vi "ProfiledPIDController_Execute.vi"(4 "PID Error Tolerance":T3={"PositionTolerance"=0.001, "VelocityTolerance"=9.9e+30}, 5 "Constraints":T1 {"MaxAcceleration" format="%16_6e"; "MaxVelocity" format="%16_6e"}, 6 "Period":dbl=0.02, 7 "PID Input Limits":T2, 8 "Reset":bool, 9 "SP-SetPoint Goal":dbl, 10 "PV-Measurement":dbl, 11 "PID Tuning":T4={"Kp"=0.0, "Ki"=0.0, "Kd"=0.0, "MaximumIntegral"=9.9e+30, "MinimumIntegral"=-9.9e+30}) -> (0 "out PID_CONTROLLER":T5={"Controller"={"Kp"=0.0, "Ki"=0.0, "Kd"=0.0, "Period"=0.0, "Max_Integral"=1.0, "Min_Integral"=-1.0, "Max_Input"=0.0, "Min_Input"=0.0, "Continuous"=FALSE, "PositionError"=0.0, "VelocityError"=0.0, "PrevError"=0.0, "TotalError"=0.0, "PositionTolerance"=0.05, "VelocityTolerance"=9.99e+35, "SetPoint"=0.0, "Kf"=0.0, "Prev_Deriv"=0.0, "Prev_Deriv 2"=0.0, "DerivativeFilter"=FALSE, "Min_Output"=-9.99e+35, "Max_Output"=9.9e+35, "Prev_F_P"=0.0, "Prev_F_P_2"=0.0, "AntiWindupActive"=FALSE, "Measurement"=0.0}, "Goal"={"Position"=0.0, "Velocity"=0.0}, "Setpoint"={"Position"=0.0, "Velocity"=0.0}, "Constraint"={"MaxVelocity"=0.0, "MaxAcceleration"=0.0}} {"Constraint"."MaxAcceleration" format="%16_6e"; "Constraint"."MaxVelocity" format="%16_6e"; "Setpoint"."Velocity" format="%16_6e"; "Setpoint"."Position" format="%16_6e"; "Goal"."Velocity" format="%16_6e"; "Goal"."Position" format="%16_6e"; "Controller"."Measurement" format="%16_6e"; "Controller"."Prev_F_P_2" format="%16_6e"; "Controller"."Prev_F_P" format="%16_6e"; "Controller"."Max_Output" format="%16_6e"; "Controller"."Min_Output" format="%16_6e"; "Controller"."Prev_Deriv 2" format="%16_6e"; "Controller"."Prev_Deriv" format="%16_6e"; "Controller"."Kf" format="%16_6e"; "Controller"."SetPoint" format="%16_6e"; "Controller"."VelocityTolerance" format="%16_6e"; "Controller"."PositionTolerance" format="%16_6e"; "Controller"."TotalError" format="%16_6e"; "Controller"."PrevError" format="%16_6e"; "Controller"."VelocityError" format="%16_6e"; "Controller"."PositionError" format="%16_6e"; "Controller"."Min_Input" format="%16_6e"; "Controller"."Max_Input" format="%16_6e"; "Controller"."Min_Integral" format="%16_6e"; "Controller"."Max_Integral" format="%16_6e"; "Controller"."Period" format="%16_6e"; "Controller"."Kd" format="%16_6e"; "Controller"."Ki" format="%16_6e"; "Controller"."Kp" format="%16_6e"}, 1 "AtSetpoint":bool, 2 "AtGoal":bool, 3 "CO-ControlOutput":dbl)   [LabVIEW 2019, in "Trajectory_Library.lvlib"]
doc: "Convience, single call, LabVIEW function. Creates and calculates the Profiled PID controller. Call this routine periodically to calculate the newest output for the provided inputs. \n \nInputs:\n - Constraints -- Trapezoid Constraint cluster contains\n - Maximum Velocity\n - Maximum Accleration\n - PID Input Limits -- (Optional) Cluster containing:\n - MaxInput -- (Default: 0)\n - MinInput -- (Default: 0)\n - Continous -- When True indicates that the input is continuous. (Default: False)\n - PID Tuning -- PID Tuning parameters containing:\n - Kp -- The proportional coefficient.\n - Ki -- The integral coefficient.\n - Kd -- The derivative coefficient.\n - Maximum Integral -- The maximum value of the integrator.\n - Minimum Integral -- The minimum value of the integrator.\n - PV-measurement -- The current measurement of the process variable. (PV)\n - SP-setpoint goal -- The new end goal setpoint of the controller. (SP)\n - Reset -- When True, causes the PID to be reset. (Default: False)\n - Period -- Period of repeated calls in seconds. (Default: 0.020)\n - PID Error Tolerance -- Tolerances for determining \"At Setpoint\", contains:\n - Position Tolerance -- (Default: 0.001)\n - Velocity Tolerance -- (Default: 9.9E+30)\nOutputs:\n - CO-ControlOutput -- Controller output (CO) \n - AtGoal -- True when PV is within the specified tolerances of the final goal SP.\n - AtSetpoint -- True when PV is within the specified tolerances of the internediate position SP.\n - Profield PID_Controller -- Updated PID_Controller data cluster"
uses:
  Trajectory_Library.lvlib
  TypeDef/PID_CONTROLLER.ctl
  TypeDef/PID_TUNING.ctl
  TypeDef/PID_INPUT_LIMITS.ctl
  TypeDef/PID_ERROR_TOLERANCE.ctl
  TypeDef/TRAPEZOID_PROFILE_STATE.ctl
  TypeDef/TRAPEZOID_PROFILE_CONSTRAINT.ctl
  TypeDef/PROFILED_PID_CONTROLLER.ctl
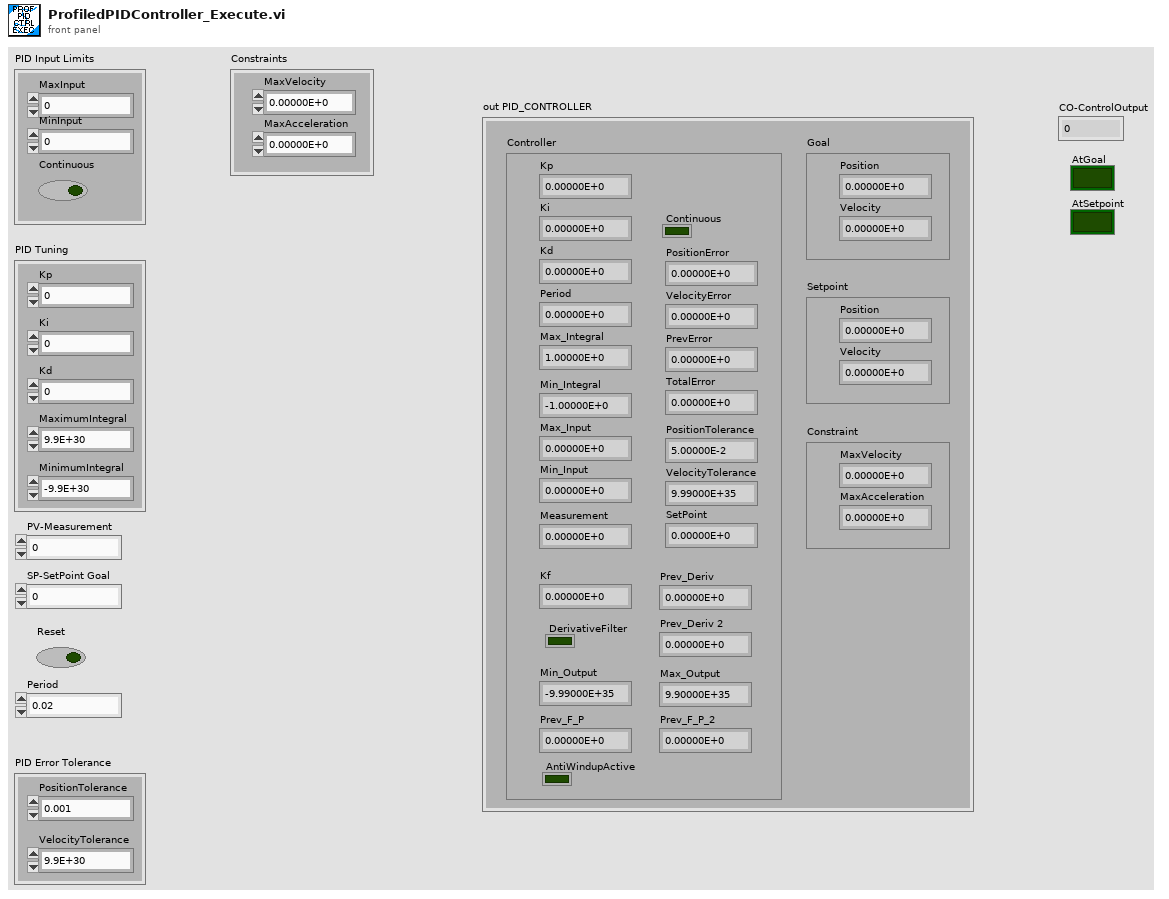
[diagram p1: front panel]
types:
  T1 = typedef "Trajectory_Library.lvlib/TRAPEZOID_PROFILE_CONSTRAINT.ctl" = cluster{"MaxVelocity":dbl, "MaxAcceleration":dbl}
  T2 = typedef "Trajectory_Library.lvlib/PID_INPUT_LIMITS.ctl" = cluster{"MaxInput":dbl, "MinInput":dbl, "Continuous":bool}
  T3 = typedef "Trajectory_Library.lvlib/PID_ERROR_TOLERANCE.ctl" = cluster{"PositionTolerance":dbl, "VelocityTolerance":dbl}
  T4 = typedef "Trajectory_Library.lvlib/PID_TUNING.ctl" = cluster{"Kp":dbl, "Ki":dbl, "Kd":dbl, "MaximumIntegral":dbl, "MinimumIntegral":dbl}
  T5 = typedef "Trajectory_Library.lvlib/PROFILED_PID_CONTROLLER.ctl" = cluster{"Controller":T6, "Goal":T7, "Setpoint":T7, "Constraint":T1}
  T6 = typedef "Trajectory_Library.lvlib/PID_CONTROLLER.ctl" = cluster{"Kp":dbl, "Ki":dbl, "Kd":dbl, "Period":dbl, "Max_Integral":dbl, "Min_Integral":dbl, "Max_Input":dbl, "Min_Input":dbl, "Continuous":bool, "PositionError":dbl, "VelocityError":dbl, "PrevError":dbl, "TotalError":dbl, "PositionTolerance":dbl, "VelocityTolerance":dbl, "SetPoint":dbl, "Kf":dbl, "Prev_Deriv":dbl, "Prev_Deriv 2":dbl, "DerivativeFilter":bool, "Min_Output":dbl, "Max_Output":dbl, "Prev_F_P":dbl, "Prev_F_P_2":dbl, "AntiWindupActive":bool, "Measurement":dbl}
  T7 = typedef "Trajectory_Library.lvlib/TRAPEZOID_PROFILE_STATE.ctl" = cluster{"Position":dbl, "Velocity":dbl}
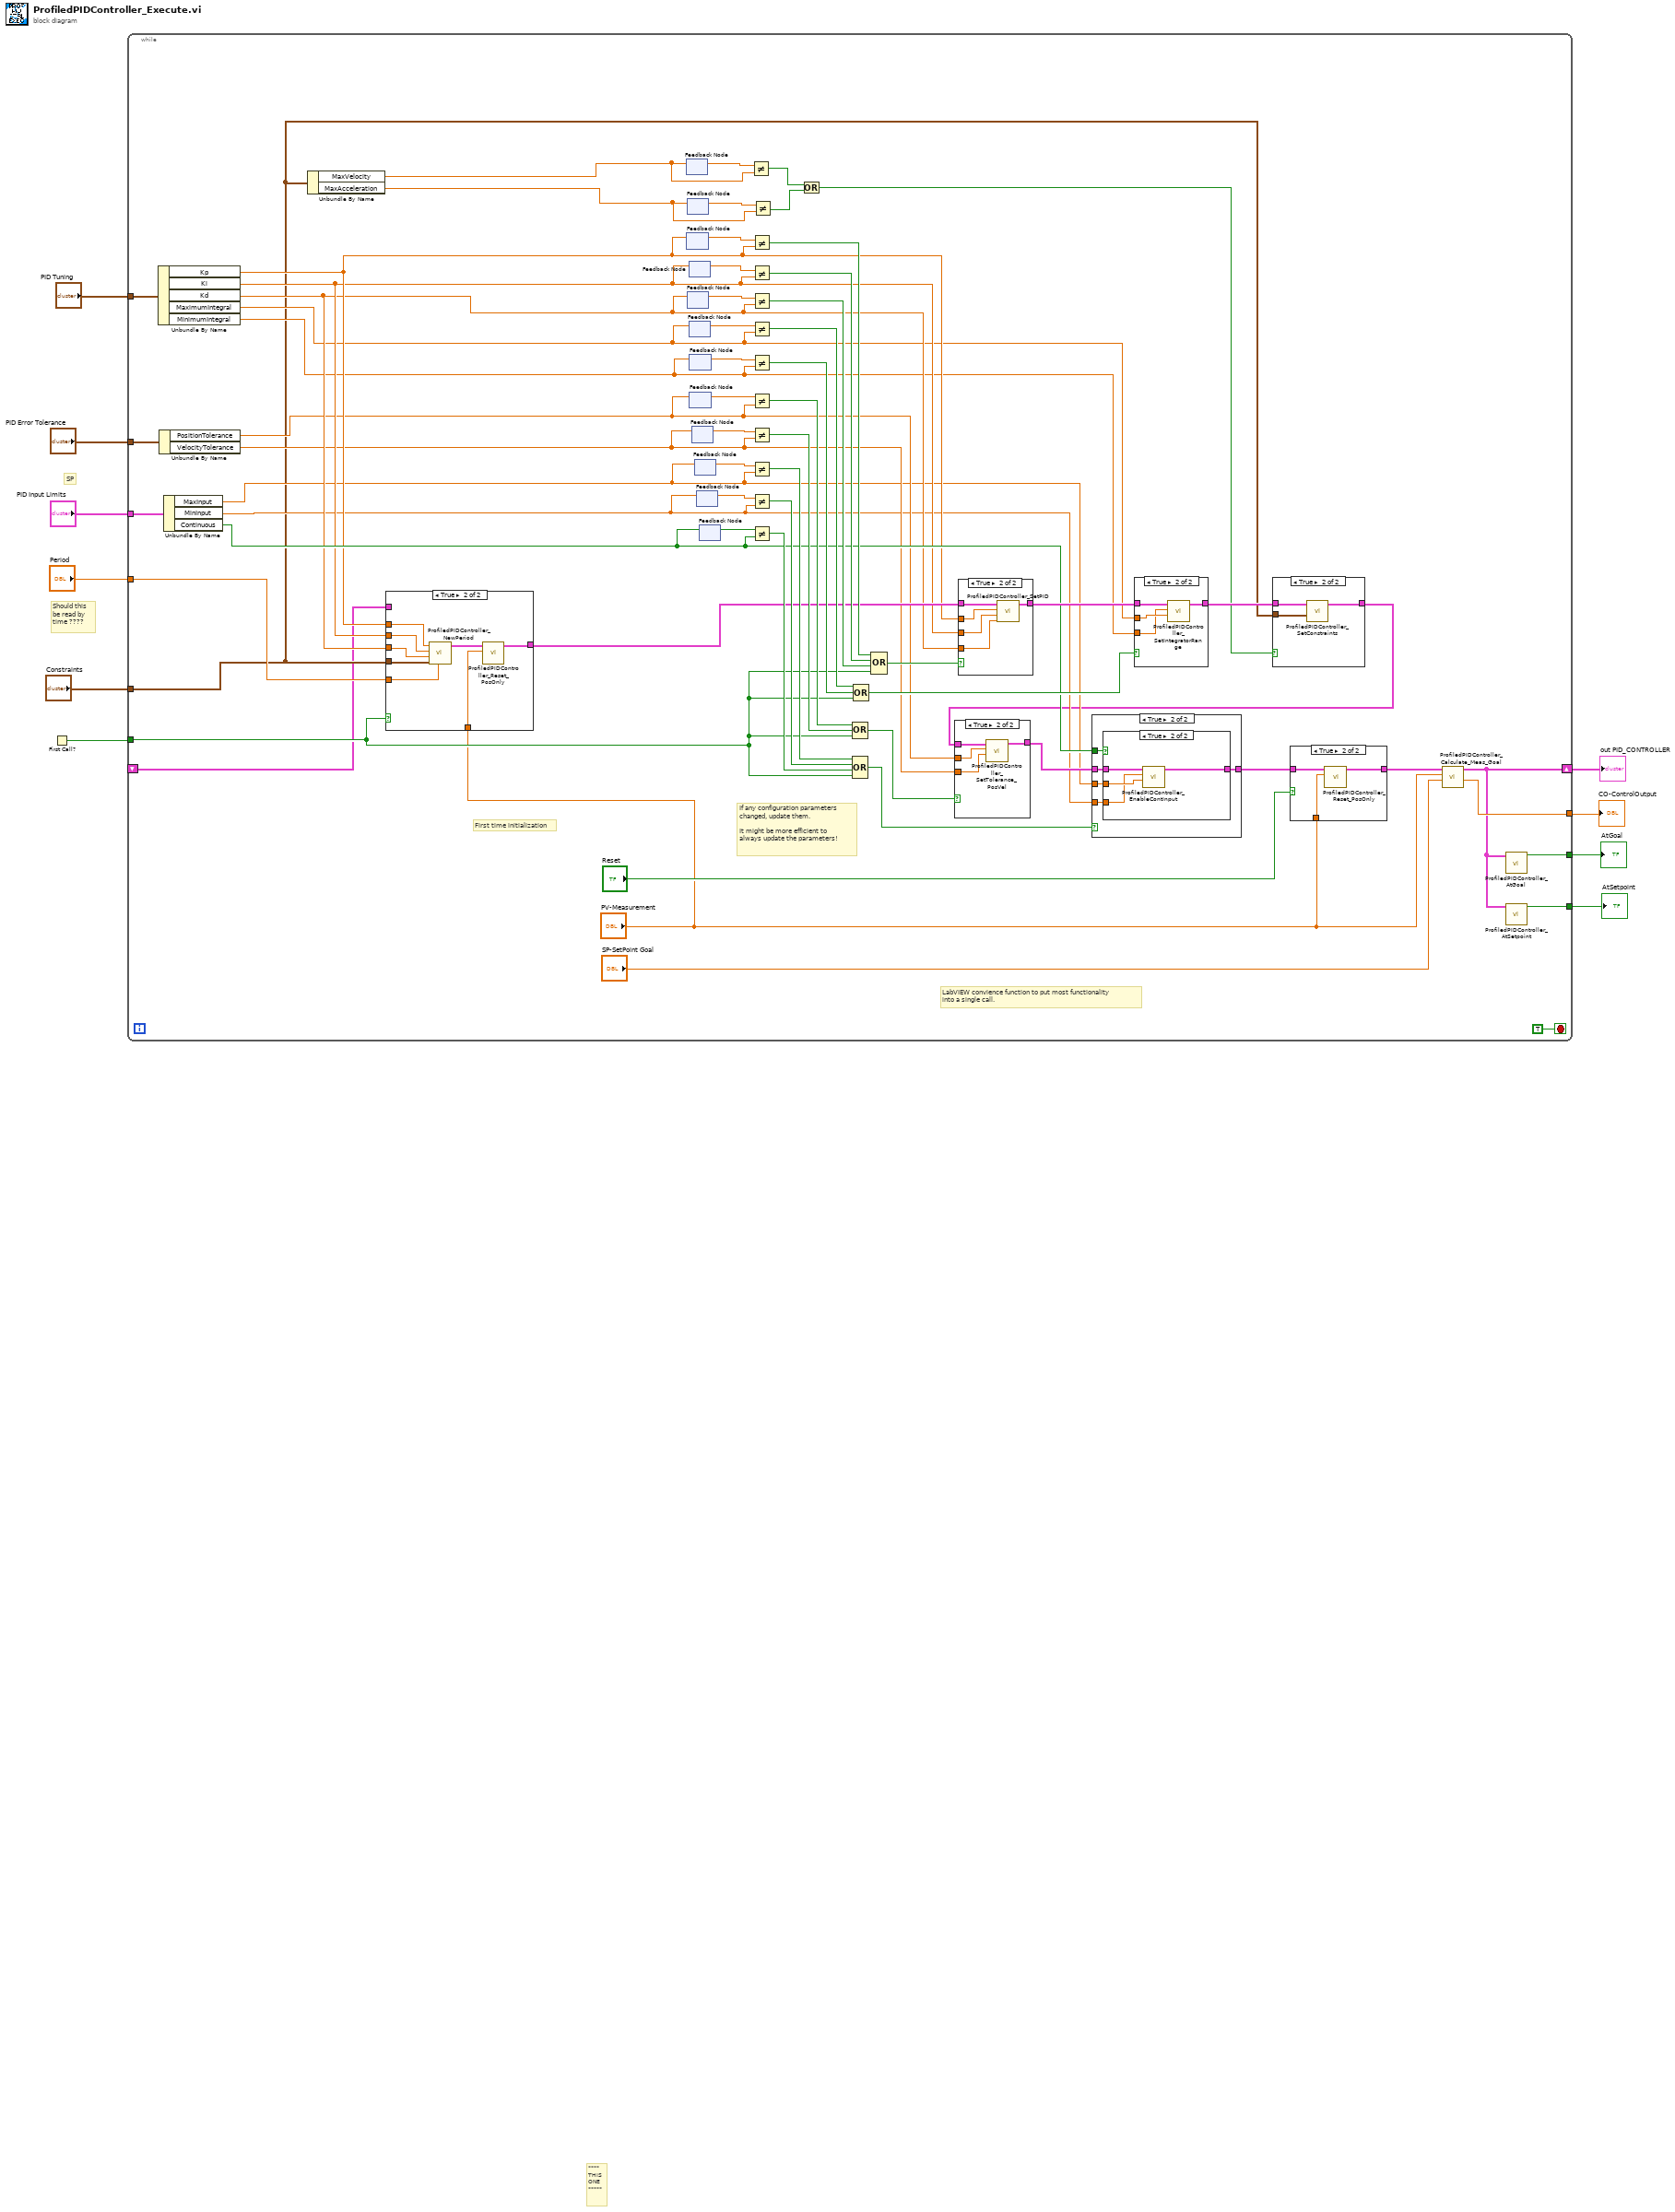
[diagram p0: block diagram]
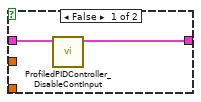
[diagram p6: hidden frame]
diagram:
  # "Should this\nbe read by\ntime ????"
  # "SP"
  # "****\nTHIS\nONE\n*****"
  n1 = First Call?() -> (First Call?: T/F=w4:bool)
  n2 = while {
    tunnel: [w73] -> w10
    tunnel: "PID Tuning" -> [w71]
    tunnel: [w70] -> w8
    tunnel: "PID Error Tolerance" -> [w69]
    tunnel: "PID Input Limits" -> [w68]
    tunnel: "Period" -> [w66]
    tunnel: w4 -> [w26]
    tunnel: [w24] -> w3
    tunnel: "Constraints" -> [w13]
    shift-right: [w23] -> w2
    shift-left: _ -> [w12]
    stop <- TRUE stop-if-true
    # "First time initialization"
    # "If any configuration parameters \nchanged, update them.\n\nIt might be more efficient to\nalways update the parameters!"
    # "LabVIEW convience function to put most functionality\ninto a single call."
    n3 = Unbundle By Name(w71) -> ("Kp"=w44:dbl, "Ki"=w43:dbl, "Kd"=w42:dbl, "MaximumIntegral"=w41:dbl, "MinimumIntegral"=w40:dbl)
    n4 = Unbundle By Name(w69) -> ("PositionTolerance"=w39:dbl, "VelocityTolerance"=w38:dbl)
    n5 = Unbundle By Name(w68) -> ("MaxInput"=w37:dbl, "MinInput"=w36:dbl, "Continuous"=w46:bool)
    n6 = Unbundle By Name(w13) -> ("MaxVelocity"=w17:dbl, "MaxAcceleration"=w18:dbl)
    n7 = case shown="True" w26 {
      tunnel: w44 -> [_ w86]
      tunnel: w43 -> [_ w85]
      tunnel: w42 -> [_ w84]
      tunnel: w66 -> [_ w83]
      tunnel: [w78 w80] -> w47
      tunnel: w12 -> [w78 _]
      tunnel: w13 -> [_ w81]
      tunnel: "PV-Measurement" -> [_ w79]
      frame False {
      }
      frame True {
        n8 = call "ProfiledPIDController_NewPeriod.vi"("Period"=w83, "Constraints"=w81, "Kd"=w84, "Ki"=w85, "Kp"=w86) -> ("PROFILED_PID_CONTROLLER"=w82:T5)  [unwired: 6 in]
        n9 = call "ProfiledPIDController_Reset_PosOnly.vi"("Position"=w79, "in PROFILED_PID_CONTROLLER"=w82) -> ("out PROFILED_PID_CONTROLLER"=w80:T5)  [unwired: 9 in]
      }
    }
    n10 = feedback #1() -> (w19:dbl)  [unwired: 1 in]
    n11 = feedback-in #1(w17) -> ()
    n12 = feedback #2() -> (w35:dbl)  [unwired: 1 in]
    n13 = feedback-in #2(w44) -> ()
    n14 = feedback #3() -> (w22:dbl)  [unwired: 1 in]
    n15 = feedback-in #3(w18) -> ()
    n16 = feedback #4() -> (w33:dbl)  [unwired: 1 in]
    n17 = feedback-in #4(w42) -> ()
    n18 = feedback #5() -> (w34:dbl)  [unwired: 1 in]
    n19 = feedback-in #5(w43) -> ()
    n20 = feedback #6() -> (w32:dbl)  [unwired: 1 in]
    n21 = feedback-in #6(w41) -> ()
    n22 = feedback #7() -> (w31:dbl)  [unwired: 1 in]
    n23 = feedback-in #7(w40) -> ()
    n24 = feedback #8() -> (w30:dbl)  [unwired: 1 in]
    n25 = feedback-in #8(w39) -> ()
    n26 = feedback #9() -> (w29:dbl)  [unwired: 1 in]
    n27 = feedback-in #9(w38) -> ()
    n28 = feedback #10() -> (w28:dbl)  [unwired: 1 in]
    n29 = feedback-in #10(w37) -> ()
    n30 = feedback #11() -> (w27:dbl)  [unwired: 1 in]
    n31 = feedback-in #11(w36) -> ()
    n32 = feedback #12() -> (w45:bool)  [unwired: 1 in]
    n33 = feedback-in #12(w46) -> ()
    n34 = Not Equal?(x=w19, y=w17) -> (x != y?=w16:bool)
    n35 = Not Equal?(x=w35, y=w44) -> (x != y?=w56:bool)
    n36 = Not Equal?(x=w34, y=w43) -> (x != y?=w57:bool)
    n37 = Not Equal?(x=w33, y=w42) -> (x != y?=w58:bool)
    n38 = Not Equal?(x=w32, y=w41) -> (x != y?=w59:bool)
    n39 = Not Equal?(x=w31, y=w40) -> (x != y?=w60:bool)
    n40 = Not Equal?(x=w30, y=w39) -> (x != y?=w61:bool)
    n41 = Not Equal?(x=w29, y=w38) -> (x != y?=w62:bool)
    n42 = Not Equal?(x=w28, y=w37) -> (x != y?=w63:bool)
    n43 = Not Equal?(x=w27, y=w36) -> (x != y?=w64:bool)
    n44 = Not Equal?(x=w45, y=w46) -> (x != y?=w65:bool)
    n45 = Not Equal?(x=w22, y=w18) -> (x != y?=w15:bool)
    n46 = Or(x=w16, y=w15) -> (x .or. y?=w14:bool)
    n47 = Compound Arithmetic op=OR(w61, w62, w26) -> (w52:bool)
    n48 = Compound Arithmetic op=OR(w63, w64, w65, w26) -> (w51:bool)
    n49 = Compound Arithmetic op=OR(w59, w60, w26) -> (w53:bool)
    n50 = Compound Arithmetic op=OR(w56, w57, w58, w26) -> (w55:bool)
    n51 = case shown="True" w55 {
      tunnel: w47 -> [w113 w118]
      tunnel: w44 -> [_ w117]
      tunnel: w43 -> [_ w116]
      tunnel: w42 -> [_ w115]
      tunnel: [w113 w114] -> w54
      frame False {
      }
      frame True {
        n52 = call "ProfiledPIDController_SetPID.vi"("Kd"=w115, "Ki"=w116, "Kp"=w117, "in PROFILED_PID_CONTROLLER"=w118) -> ("out PROFILED_PID_CONTROLLER"=w114:T5)  [unwired: 7 in]
      }
    }
    n53 = case shown="True" w53 {
      tunnel: w54 -> [w108 w112]
      tunnel: w41 -> [_ w111]
      tunnel: w40 -> [_ w110]
      tunnel: [w108 w109] -> w21
      frame False {
      }
      frame True {
        n54 = call "ProfiledPIDController_SetIntegratorRange.vi"("Maximum"=w111, "Minimum"=w110, "in PROFILED_PID_CONTROLLER"=w112) -> ("out PROFILED_PID_CONTROLLER"=w109:T5)  [unwired: 8 in]
      }
    }
    n55 = case shown="True" w14 {
      tunnel: w21 -> [w74 w77]
      tunnel: [w74 w76] -> w20
      tunnel: w13 -> [_ w75]
      frame False {
      }
      frame True {
        n56 = call "ProfiledPIDController_SetConstraints.vi"("Constraint"=w75, "in PROFILED_PID_CONTROLLER"=w77) -> ("out PROFILED_PID_CONTROLLER"=w76:T5)  [unwired: 9 in]
      }
    }
    n57 = case shown="True" w52 {
      tunnel: w20 -> [w103 w107]
      tunnel: w39 -> [_ w106]
      tunnel: w38 -> [_ w105]
      tunnel: [w103 w104] -> w50
      frame False {
      }
      frame True {
        n58 = call "ProfiledPIDController_SetTolerance_PosVel.vi"("VelocityTolerance"=w105, "PositionTolerance"=w106, "in PROFILED_PID_CONTROLLER"=w107) -> ("out PROFILED_PID_CONTROLLER"=w104:T5)  [unwired: 8 in]
      }
    }
    n59 = case shown="True" w51 {
      tunnel: w37 -> [_ w96]
      tunnel: w36 -> [_ w95]
      tunnel: w50 -> [w91 w94]
      tunnel: w46 -> [_ w93]
      tunnel: [w91 w92] -> w49
      frame False {
      }
      frame True {
        n60 = case shown="True" w93 {
          tunnel: w94 -> [w98 w102]
          tunnel: [w97 w101] -> w92
          tunnel: w96 -> [_ w100]
          tunnel: w95 -> [_ w99]
          frame False {
            n61 = call "ProfiledPIDController_DisableContInput.vi"("in PROFILED_PID_CONTROLLER"=w98) -> ("out PROFILED_PID_CONTROLLER"=w97:T5)  [unwired: 10 in]
          }
          frame True {
            n62 = call "ProfiledPIDController_EnableContInput.vi"("MaxInput"=w100, "MinInput"=w99, "in PROFILED_PID_CONTROLLER"=w102) -> ("out PROFILED_PID_CONTROLLER"=w101:T5)  [unwired: 8 in]
          }
        }
      }
    }
    n63 = case shown="True" "Reset" {
      tunnel: w49 -> [w87 w90]
      tunnel: [w87 w89] -> w48
      tunnel: "PV-Measurement" -> [_ w88]
      frame False {
      }
      frame True {
        n64 = call "ProfiledPIDController_Reset_PosOnly.vi"("Position"=w88, "in PROFILED_PID_CONTROLLER"=w90) -> ("out PROFILED_PID_CONTROLLER"=w89:T5)  [unwired: 9 in]
      }
    }
    n65 = call "ProfiledPIDController_Calculate_Meas_Goal.vi"("SP-Goal"="SP-SetPoint Goal", "PV-Measurement"="PV-Measurement", "in PROFILED_PID_CONTROLLER"=w48) -> ("CO-ControlOutput"=w73:dbl, "out PROFILED_PID_CONTROLLER"=w23:T5)  [unwired: 7 in]
    n66 = call "ProfiledPIDController_AtGoal.vi"("in PROFILED_PID_CONTROLLER"=w23) -> ("AtGoal"=w70:bool)  [unwired: 10 in]
    n67 = call "ProfiledPIDController_AtSetpoint.vi"("in PROFILED_PID_CONTROLLER"=w23) -> ("AtSetpoint"=w24:bool)  [unwired: 10 in]
  }
  "out PID_CONTROLLER" <- w2
  "CO-ControlOutput" <- w10
  "AtGoal" <- w8
  "AtSetpoint" <- w3
